vi "Enable Caching.vi"(8 "error in (no error)":errorcluster, 10 "Server Caching":T1={"Auto Cache Static Files"=TRUE, "Cache Folder"=path "", "Memory Caching Bytes Limit"=0, "Memory Caching Age Limit"=0.0, "File Caching Age Limit"=0.0, "Default Cache Max Age"=0}, 11 "Server in":refnum<class "Server.lvclass">) -> (0 "error out":errorcluster, 3 "Server out":refnum<class "Server.lvclass">)   [LabVIEW 2020, in "HTTP Server.lvlib" / "Server.lvclass"]
doc: "<b>Caching is currently broken!</b>\n\nProvides mechanisms for keeping sufficiently small, frequently requested files in memory for faster serving as well as persisting programmatically generated responses to memory or disk to avoid running the generation logic again when input state hasn't changed."
uses:
  Server.lvclass
  Server Caching.ctl
  Caching Request/Caching Request.lvclass
  C:/dev/lv/2020/lv-http-server/HTTP Server/Handler/Handler.lvclass
  Caching Response/Caching Response.lvclass
  Caching Complete/Caching Complete.lvclass
  Caching/Caching.lvclass
  C:/dev/lv/2020/lv-http-server/HTTP Server/Service/Service.lvclass
  Add Connection Handler.vi
  Add Request Handler.vi
  Add Route Handler.vi
  Add Controller Handler.vi
  Add Controller.vi
  Add Response Handler.vi
  Add Complete Handler.vi
  Add Exception Handler.vi
  Connection Handler/Connection Handler.lvclass
  Request Handler/Request Handler.lvclass
  Route Handler/Route Handler.lvclass
  Controller Handler/Controller Handler.lvclass
  Controller/Controller.lvclass
  Response Handler/Response Handler.lvclass
  Complete Handler/Complete Handler.lvclass
  Exception Handler/Exception Handler.lvclass
  Handler/Handler.lvclass
  HTTP Server.lvlib
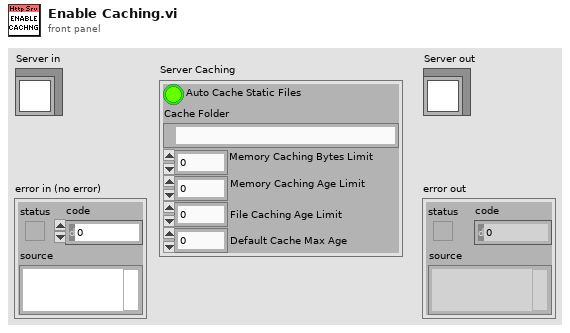
[diagram p1: front panel]
types:
  T1 = typedef "HTTP Server.lvlib/Server Caching.ctl" = cluster{"Auto Cache Static Files":bool, "Cache Folder":path, "Memory Caching Bytes Limit":i32, "Memory Caching Age Limit":dbl, "File Caching Age Limit":dbl, "Default Cache Max Age":i32}
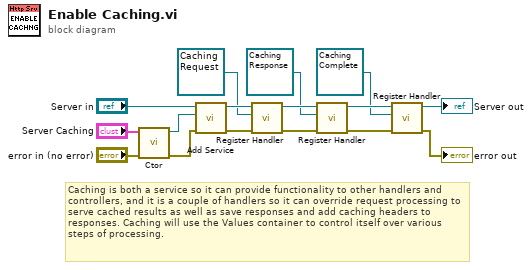
[diagram p0: block diagram]
diagram:
  # "Caching is both a service so it can provide functionality to other handlers and controllers, and it is a couple of handlers so it can override request processing to serve cached results as well as save responses and add caching headers to responses. Caching will use the Values container to control itself over various steps of processing."
  n1 = call "Ctor.vi"("error in (no error)"="error in (no error)", "Server Caching"="Server Caching") -> ("error out"=w13:errorcluster, "Caching out"=w12:refnum<class "Caching.lvclass">)  [unwired: 8 in]
  n2 = call "Add Service.vi"("error in (no error)"=w13, "Service"=w12, "Server in"="Server in") -> ("error out"=w10:errorcluster, "Server out"=w11:refnum<class "Server.lvclass">)  [unwired: 7 in]
  n3 = call "Register Handler.vi"("error in (no error)"=w10, "Handler"=refnum<class "Caching Request.lvclass"> refnum ("HTTP Server.lvlib:Caching Request.lvclass"), "Server in"=w11) -> ("error out"=w9:errorcluster, "Server out"=w8:refnum<class "Server.lvclass">)  [unwired: 7 in]
  n4 = call "Register Handler.vi"("error in (no error)"=w9, "Handler"=refnum<class "Caching Response.lvclass"> refnum ("HTTP Server.lvlib:Caching Response.lvclass"), "Server in"=w8) -> ("error out"=w6:errorcluster, "Server out"=w7:refnum<class "Server.lvclass">)  [unwired: 7 in]
  n5 = call "Register Handler.vi"("error in (no error)"=w6, "Handler"=refnum<class "Caching Complete.lvclass"> refnum ("HTTP Server.lvlib:Caching Complete.lvclass"), "Server in"=w7) -> ("error out"=→"error out":errorcluster, "Server out"=→"Server out":refnum<class "Server.lvclass">)  [unwired: 7 in]
